vi "Home.vi"() -> ()   [LabVIEW 2019]
uses:
  <vilib>/NI/Current Value Table/Type Defs/Single Tag.ctl
  <vilib>/NI/Current Value Table/Type Defs/Data Types.ctl
  <vilib>/NI/STM/TCP/Read Meta Data (TCP Ref).vi
  <vilib>/NI/STM/TCP/Get Connection Reference (TCP).vi
  <vilib>/NI/AMC/Read Termination Message.vi
  <vilib>/NI/AMC/Create Single Message.vi
  <vilib>/NI/AMC/Update Message Routing Info.vi
  <vilib>/NI/STM/TCP/Read Meta Data (TCP Clst).vi
  <vilib>/NI/AMC/Globals.vi
  <vilib>/NI/STM/TCP/Write Message (TCP).vi
  <vilib>/NI/AMC/Send Message.vi
  <vilib>/NI/AMC/AMC.lvlib
  <vilib>/NI/STM/NI STM.lvlib
  <vilib>/NI/Current Value Table/Current Value Table.lvlib
panel:
  in  "Reset Alarms":bool
  in  "Run":bool
  in  "Alarms":i32(listbox)=-1
  out "PLC Model":string
  out "PLC Firmware":string
  out "PLC Sweep Time":dbl format="%#.4f"
  in  "Exit":bool
  in  "Dosing":bool
  in  "Mixing Tank":bool
  in  "Process 3":bool
  in  "Process 2":bool
  in  "Process 1":bool
  out "status":string
  in  "Home Btn":bool
  in  "Facilities Btn":bool
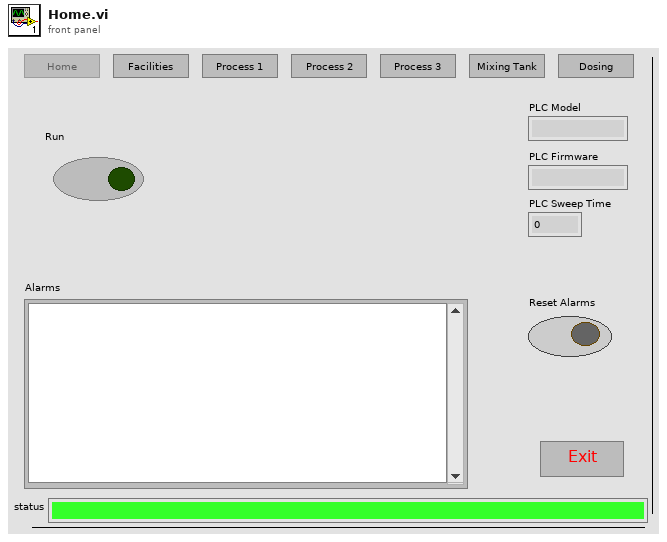
[diagram p1: front panel]
types:
  T1 = typedef "Current Value Table.lvlib/Single Tag.ctl" = cluster{"Data Type":T2, "Name":string, "Value":string, "Description":string}
  T2 = typedef "Current Value Table.lvlib/Data Types.ctl" = enum16{"Double", "Single", "I64", "I32", "I16", "I8", "U64", "U32", "U16", "U8", "String", "Boolean", "Array of U8", "Array of U16", "Array of U32", "Array of U64", "Array of I64", "Array of I32", "Array of I16", "Array of I8", "Array of Double", "Array of Single", "Array of Boolean", "Array of String"}
  T3 = typedef "AMC.lvlib/Message Queue.ctl" = refnum<queue>
  T4 = typedef "NI STM.lvlib/TCP Connection Info.ctl" = cluster{"connection ID":refnum<k5>, "meta data":T5[]}
  T5 = typedef "NI STM.lvlib/MetaDataElement.ctl" = string
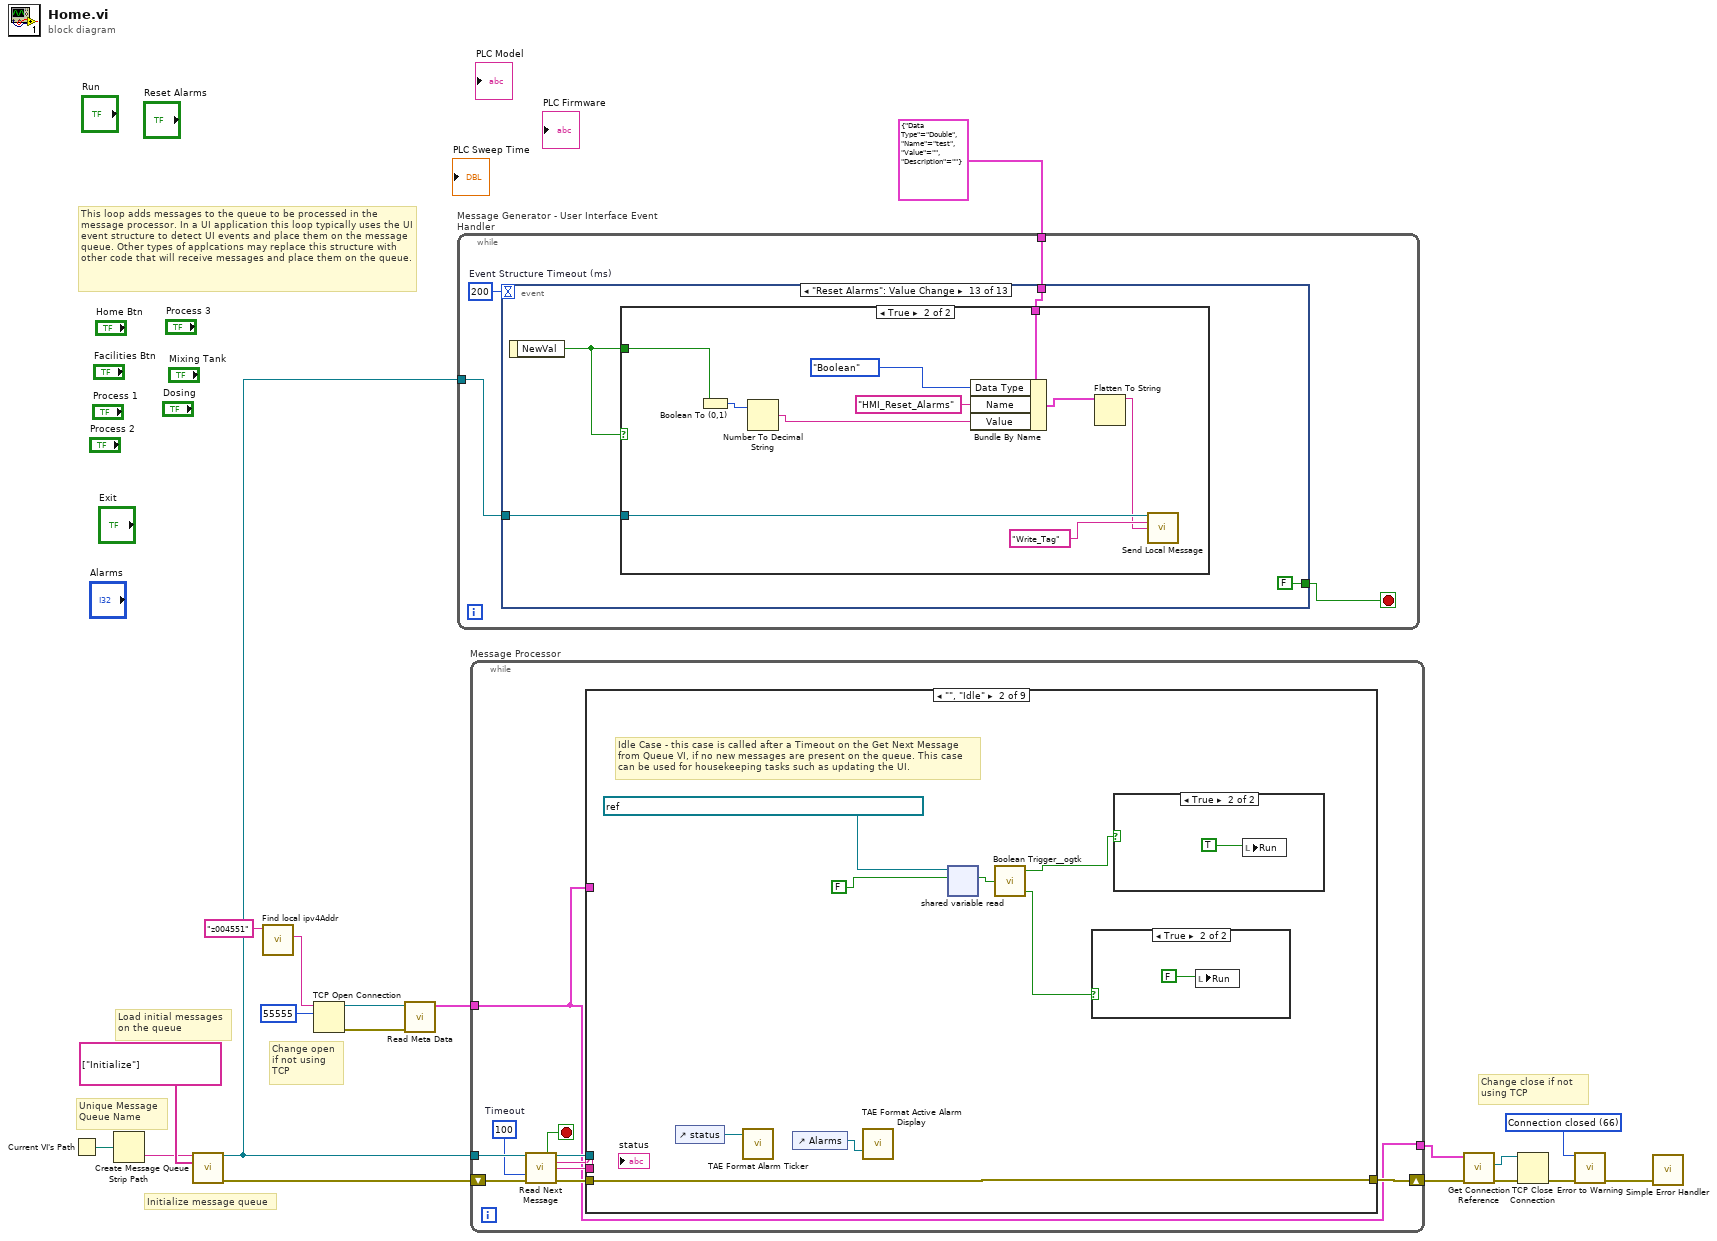
[diagram p0: block diagram]
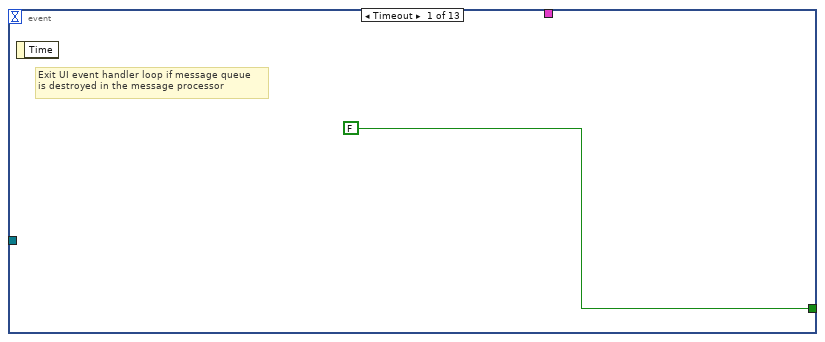
[diagram p2: hidden frame]
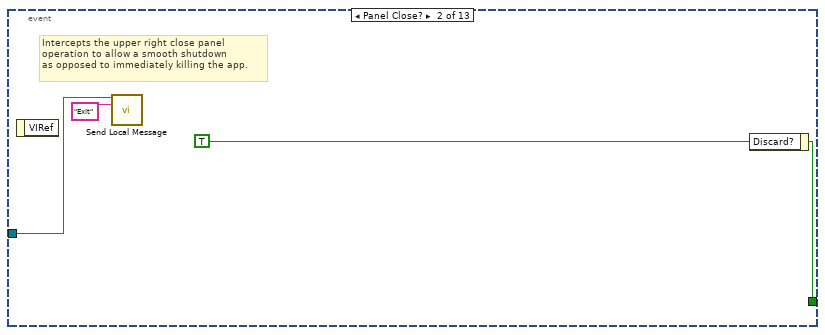
[diagram p3: hidden frame]
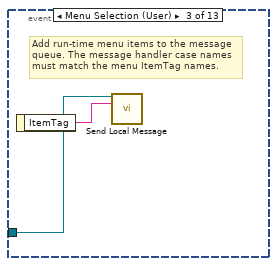
[diagram p4: hidden frame]
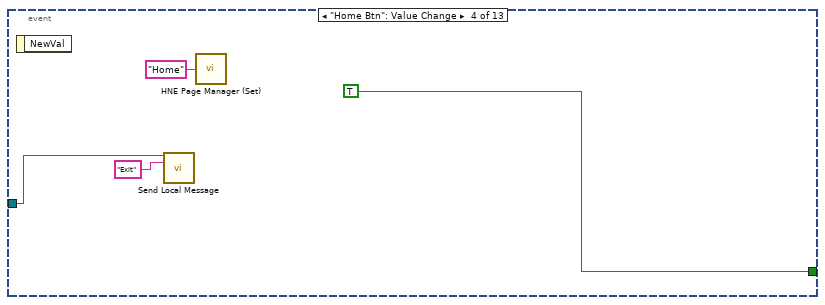
[diagram p5: hidden frame]
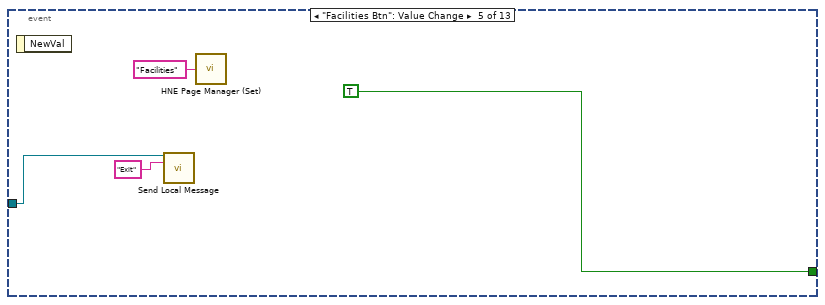
[diagram p6: hidden frame]
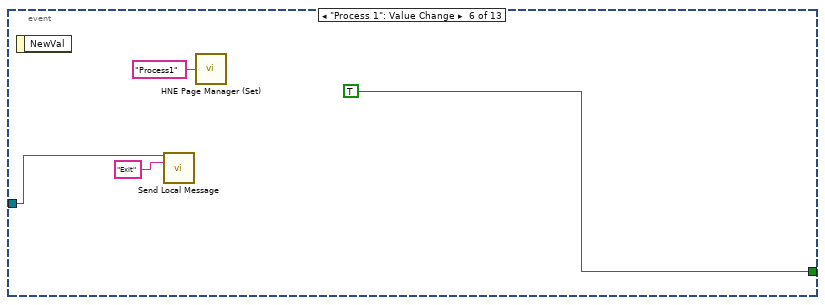
[diagram p7: hidden frame]
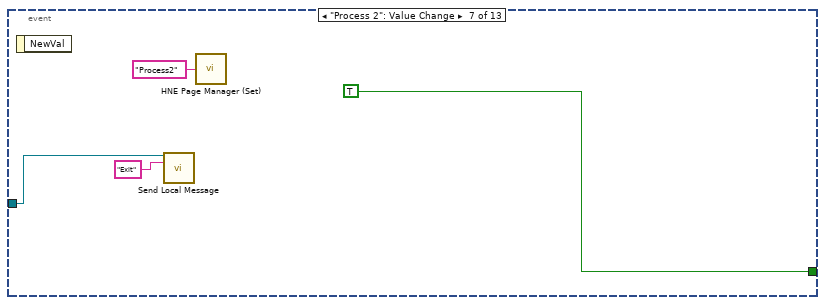
[diagram p8: hidden frame]
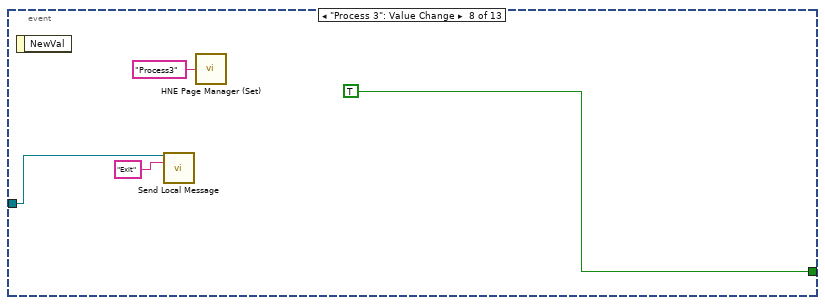
[diagram p9: hidden frame]
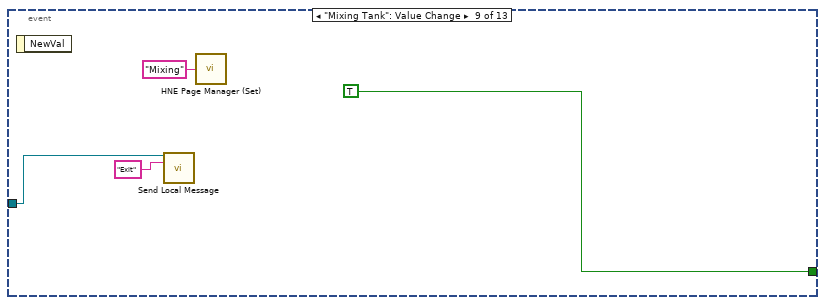
[diagram p10: hidden frame]
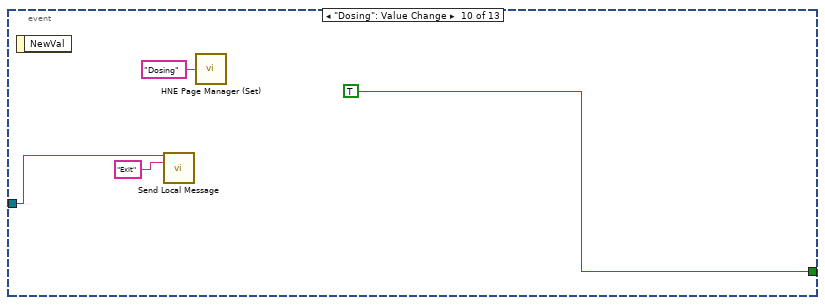
[diagram p11: hidden frame]
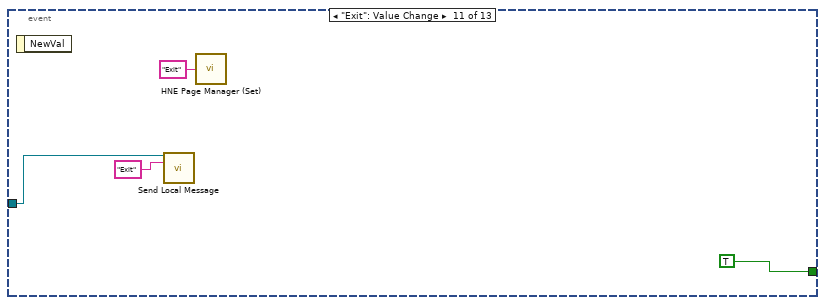
[diagram p12: hidden frame]
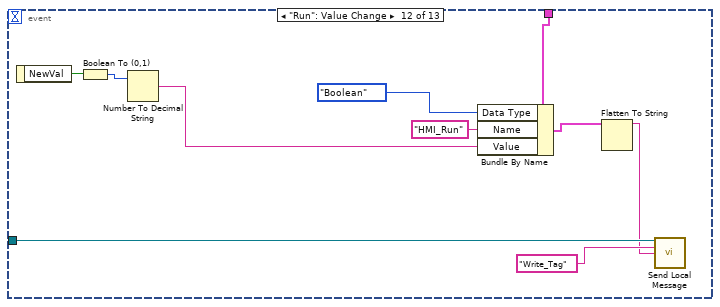
[diagram p13: hidden frame]
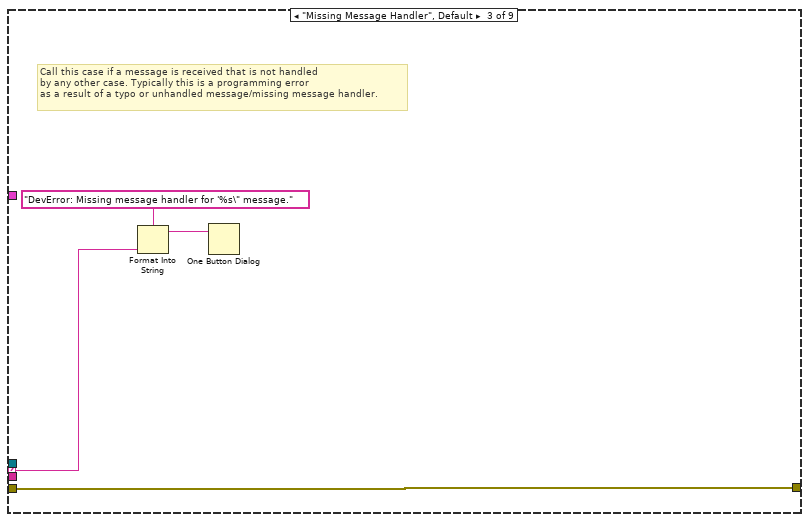
[diagram p18: hidden frame]
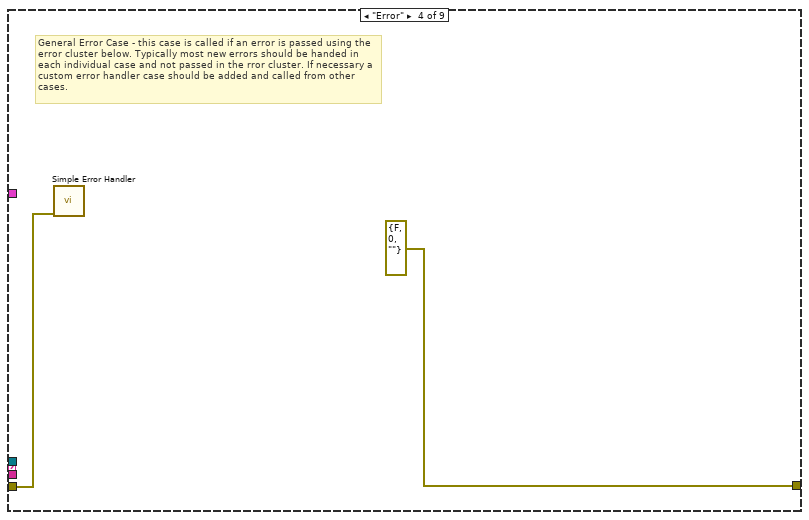
[diagram p19: hidden frame]
diagram:
  w8 = 66 items=["No Error", "Argument Error", "Memory Full", "Out of Zone", "End of File", "File Already Open", "Generic File IO Error", "File Not Found", "File Permission Error", "Disk Full", "Duplicate Path", "Too Many Files Open", "Not Enabled", "Resource File Not Found", "Cannot Add Resource", "Resource Not Found", "Image Not Found", "Image Memory Error", "Pen Does Not Exist", "Config Bad Type", "Config Token Not Found", "Config Parse Error", "Config Memory Error", "Bad External Code Format", "Bad External Code Offset", "External Code Not Present", "Null Window", "Destroy Window Mixup", "Null Menu", "Print Aborted", "Bad Print Record", "Print Driver Error", "Windows Error During Print", "Memory Error During Print", "Print Dialog Error", "Generic Print Error", "Invalid Device Refnum", "Device Not Found", "Device Parameter Error", "Device Unit Error", "Can't Open Device", "Device Call Aborted", "Generic Error", "Cancelled By User", "Object ID Too Low", "Object ID Too High", "Object Not In Heap", "Unknown Heap", "Bad DefProc ID", "DefProc Not In Table", "Message Out Of Range", "Null Method", "Unknown Message", "Manager Call Not Supported", "Bad address", "Connection In progress", "Connection timed out", "Connection is already in progress", "Network attribute not supported", "Network error", "Address in use", "System out of memory", "Connection aborted", "Connection refused", "Connection is not connected", "Connection is already connected", "Connection closed", "Initialize error (interapplication manager)", "Bad occurrence", "Wait on unbound occurrence handler", "Occurrence queue overflow", "Bad path", "Semaphore not signaled", "Unrecognized type (interapplication manager)"] ("1st Error to Convert")
  # "Change close if not using TCP"
  # "Change open if not using TCP"
  # "This loop adds messages to the queue to be processed in the message processor. In a UI application this loop typically uses the UI event structure to detect UI events and place them on the message queue. Other types of applcations may replace this structure with other code that will receive messages and place them on the queue."
  # "Initialize message queue"
  # "Unique Message\nQueue Name"
  # "Load initial messages\non the queue"
  n1 = Current VI's Path() -> (path=w15:path)
  n2 = Strip Path(path=w15) -> (name=w18:string)  [unwired: 1 out]
  n3 = call <vilib>:"Create Message Queue.vi"("message queue name"=w18, "initial message names"=string[] ["Initialize"]) -> ("message queue out"=w17:T3, "error out"=w16:errorcluster)  [unwired: 12 in]
  n4 = call "Find local ipv4Addr.vi"("MachineToFind"="z004551") -> ("name"=w11:string)  [unwired: 9 in, 1 out]
  n5 = TCP Open Connection(address=w11, remote port or service name=u16 55555 ("remote port")) -> (connection ID=w13:refnum<k5>, error out=w12:errorcluster)  [unwired: 1 in, 2 out]
  n6 = call-poly <vilib>:"Read Meta Data.vi"("error in"=w12, "connection ID"=w13) -> ("connection info out"=w3:T4)  [unwired: 7 in, 2 out]
  n7 = while "Message Generator - User Interface Event Handler" {
    tunnel: w17 -> [w21]
    tunnel: T1 {"Data Type"=enum."Double", "Name"="test", "Value"="", "Description"=""} ("Tag") -> [w20]
    stop <- w22 stop-if-true
    w23 = 200  # Event Structure Timeout (ms)
    n8 = event shown="[12] \"Reset Alarms\": Value Change" {
      selector: _ -> [_ _ _ _ _ _ _ _ _ _ _ _ _]
      dyn-events: _ -> [_ _ _ _ _ _ _ _ _ _ _ _ _]
      timeout: w23 -> [_ _ _ _ _ _ _ _ _ _ _ _ _]
      tunnel: [FALSE ("Discard?") w27 _ TRUE ("Discard?") TRUE ("Discard?") TRUE ("Discard?") TRUE ("Discard?") TRUE ("Discard?") TRUE ("Discard?") TRUE ("Discard?") TRUE ("Discard?") _ FALSE ("Discard?")] -> w22
      tunnel: w21 -> [_ w25 w28 w30 w34 w38 w42 w46 w50 w54 w58 w71 w75]
      tunnel: w20 -> [_ _ _ _ _ _ _ _ _ _ _ w67 w74]
      event Timeout {
        # "Exit UI event handler loop if message queue\nis destroyed in the message processor"
        n9 = event-data() -> ()  [unwired: 2 out]
      }
      event Panel Close? {
        w27 = TRUE ("Discard?")
        # "Intercepts the upper right close panel\noperation to allow a smooth shutdown\nas opposed to immediately killing the app."
        n10 = event-data() -> ()  [unwired: 2 out]
        n11 = call <vilib>:"Send Local Message.vi"("message queue in"=w25, "message name"="Exit") -> ()  [unwired: 11 in, 3 out]
        n12 = event-data("Discard?"=w27) -> ()  [unwired: 1 in, 1 out]
      }
      event Menu Selection (User) {
        # "Add run-time menu items to the message\nqueue. The message handler case names must match the menu ItemTag names."
        n13 = event-data() -> ("ItemTag"=w29:string)  [unwired: 1 out]
        n14 = call <vilib>:"Send Local Message.vi"("message queue in"=w28, "message name"=w29) -> ()  [unwired: 11 in, 3 out]
      }
      event "Home Btn": Value Change {
        n15 = event-data() -> ()  [unwired: 2 out]
        n16 = call <vilib>:"Send Local Message.vi"("message queue in"=w30, "message name"="Exit") -> ()  [unwired: 11 in, 3 out]
        n17 = call <userlib>:"HNE Page Manager (Set).vi"("Next Page"="Home") -> ()  [unwired: 4 in, 1 out]
      }
      event "Facilities Btn": Value Change {
        n18 = event-data() -> ()  [unwired: 2 out]
        n19 = call <vilib>:"Send Local Message.vi"("message queue in"=w34, "message name"="Exit") -> ()  [unwired: 11 in, 3 out]
        n20 = call <userlib>:"HNE Page Manager (Set).vi"("Next Page"="Facilities") -> ()  [unwired: 4 in, 1 out]
      }
      event "Process 1": Value Change {
        n21 = event-data() -> ()  [unwired: 2 out]
        n22 = call <vilib>:"Send Local Message.vi"("message queue in"=w38, "message name"="Exit") -> ()  [unwired: 11 in, 3 out]
        n23 = call <userlib>:"HNE Page Manager (Set).vi"("Next Page"="Process1") -> ()  [unwired: 4 in, 1 out]
      }
      event "Process 2": Value Change {
        n24 = event-data() -> ()  [unwired: 2 out]
        n25 = call <vilib>:"Send Local Message.vi"("message queue in"=w42, "message name"="Exit") -> ()  [unwired: 11 in, 3 out]
        n26 = call <userlib>:"HNE Page Manager (Set).vi"("Next Page"="Process2") -> ()  [unwired: 4 in, 1 out]
      }
      event "Process 3": Value Change {
        n27 = event-data() -> ()  [unwired: 2 out]
        n28 = call <vilib>:"Send Local Message.vi"("message queue in"=w46, "message name"="Exit") -> ()  [unwired: 11 in, 3 out]
        n29 = call <userlib>:"HNE Page Manager (Set).vi"("Next Page"="Process3") -> ()  [unwired: 4 in, 1 out]
      }
      event "Mixing Tank": Value Change {
        n30 = event-data() -> ()  [unwired: 2 out]
        n31 = call <vilib>:"Send Local Message.vi"("message queue in"=w50, "message name"="Exit") -> ()  [unwired: 11 in, 3 out]
        n32 = call <userlib>:"HNE Page Manager (Set).vi"("Next Page"="Mixing") -> ()  [unwired: 4 in, 1 out]
      }
      event "Dosing": Value Change {
        n33 = event-data() -> ()  [unwired: 2 out]
        n34 = call <vilib>:"Send Local Message.vi"("message queue in"=w54, "message name"="Exit") -> ()  [unwired: 11 in, 3 out]
        n35 = call <userlib>:"HNE Page Manager (Set).vi"("Next Page"="Dosing") -> ()  [unwired: 4 in, 1 out]
      }
      event "Exit": Value Change {
        n36 = event-data() -> ()  [unwired: 2 out]
        n37 = call <vilib>:"Send Local Message.vi"("message queue in"=w58, "message name"="Exit") -> ()  [unwired: 11 in, 3 out]
        n38 = call <userlib>:"HNE Page Manager (Set).vi"("Next Page"="Exit") -> ()  [unwired: 4 in, 1 out]
      }
      event "Run": Value Change {
        n39 = event-data() -> ("NewVal"=w69:bool)  [unwired: 1 out]
        n40 = Boolean To (0,1)(Boolean=w69) -> (0, 1=w68:i16)
        n41 = Number To Decimal String(number=w68) -> (decimal integer string=w64:string)  [unwired: 1 in]
        n42 = Bundle By Name(cluster=w67, "Data Type"=Data_Types."Boolean", "Name"="HMI_Run", "Value"=w64) -> (w66:T1)
        n43 = Flatten To String(anything=w66) -> (data string=w65:string)  [unwired: 3 in, 2 out]
        n44 = call <vilib>:"Send Local Message.vi"("message queue in"=w71, "message name"="Write_Tag", "message value"=w65) -> ()  [unwired: 10 in, 3 out]
      }
      event "Reset Alarms": Value Change {
        n45 = event-data() -> ("NewVal"=w72:bool)  [unwired: 1 out]
        n46 = case shown="True" w72 {
          tunnel: w75 -> [_ w85]
          tunnel: w72 -> [_ w83]
          tunnel: w74 -> [_ w81]
          frame False {
          }
          frame True {
            n47 = Boolean To (0,1)(Boolean=w83) -> (0, 1=w82:i16)
            n48 = Number To Decimal String(number=w82) -> (decimal integer string=w78:string)  [unwired: 1 in]
            n49 = Bundle By Name(cluster=w81, "Data Type"=Data_Types."Boolean", "Name"="HMI_Reset_Alarms", "Value"=w78) -> (w80:T1)
            n50 = Flatten To String(anything=w80) -> (data string=w79:string)  [unwired: 3 in, 2 out]
            n51 = call <vilib>:"Send Local Message.vi"("message queue in"=w85, "message name"="Write_Tag", "message value"=w79) -> ()  [unwired: 10 in, 3 out]
          }
        }
      }
    }
  }
  n52 = while "Message Processor" {
    shift-left: w16 -> [w91]
    shift-right: [w95] -> w4
    tunnel: w17 -> [w92]
    tunnel: [w86] -> w2
    tunnel: w3 -> [w86]
    stop <- w94 stop-if-true
    w87 = 100  # Timeout
    n53 = call <vilib>:"Read Next Message.vi"("message queue in"=w92, "timeout (1 ms)"=w87, "error in"=w91) -> ("exit process?"=w94:bool, "message queue out"=w93:T3, "message name"=w89:string, "message value"=w88:string, "error out"=w90:errorcluster)  [unwired: 5 in, 3 out]
    n54 = case shown="\"\", \"Idle\"" w89 {
      selector: w89 -> [_ _ w109 _ _ _ _ _ _]
      tunnel: w93 -> [_ _ _ _ _ _ w119 _ _]
      tunnel: w90 -> [w96 w104 w110 w111 w113 w117 w120 w122 w124]
      tunnel: [w96 w104 w110 errorcluster {"status"=FALSE, "code"=0, "source"=""} ("error out") w113 w117 w118 w122 w123] -> w95
      tunnel: w88 -> [_ _ _ _ _ _ _ _ w125]
      tunnel: w86 -> [_ _ _ _ _ _ _ _ w126]
      frame "---------- Framework Operations ----------" {
        # "Dummy case to add a seperator in the Case Structure menu"
      }
      frame "", "Idle" {
        # "Idle Case - this case is called after a Timeout on the Get Next Message from Queue VI, if no new messages are present on the queue. This case can be used for housekeeping tasks such as updating the UI."
        n55 = control-ref of="status"() -> (w103:refnum<vi>)
        n56 = call <userlib>:"TAE Format Alarm Ticker.vi"("Alarm Ticker Ref"=w103) -> ()  [unwired: 15 in]
        n57 = control-ref of="Alarms"() -> (w102:refnum<vi>)
        n58 = call <userlib>:"TAE Format Active Alarm Display.vi"("List Box Ref"=w102) -> ()  [unwired: 14 in, 1 out]
        n59 = shared-variable-read(refnum<k21> "ni.var.psp://z004551/CDL0100 ReadWriteTags/HMI_Run" ("shared variable refnum in"), FALSE) -> (w99:bool)  [unwired: 1 in, 3 out]
        n60 = call <userlib>:"Boolean Trigger__ogtk.vi"("Boolean Input"=w99) -> ("Rising Edge"=w97:bool, "Falling Edge"=w98:bool)  [unwired: 1 in]
        n61 = case shown="True" w98 {
          frame False {
          }
          frame True {
            n62 = local write "Run"(FALSE) -> ()
          }
        }
        n63 = case shown="True" w97 {
          frame False {
          }
          frame True {
            n64 = local write "Run"(TRUE) -> ()
          }
        }
      }
      frame "Missing Message Handler", Default {
        # "Call this case if a message is received that is not handled \nby any other case. Typically this is a programming error\nas a result of a typo or unhandled message/missing message handler."
        n65 = Format Into String(format string="DevError: Missing message handler for '%s\" message." ("message"), w109) -> (resulting string=w107:string)  [unwired: 2 in, 1 out]
        n66 = One Button Dialog(message=w107) -> ()  [unwired: 2 out]
      }
      frame "Error" {
        # "General Error Case - this case is called if an error is passed using the error cluster below. Typically most new errors should be handed in each individual case and not passed in the rror cluster. If necessary a custom error handler case should be added and called from other cases."
        n67 = call <vilib>:"Simple Error Handler.vi"("error in (no error)"=w111) -> ()  [unwired: 1 in, 8 out]
      }
      frame "---------- Generic Operations ----------" {
        # "Dummy case to add a seperator in the Case Structure menu"
      }
      frame "Initialize" {
        # "Initialize the state variables and user interface"
        n68 = shared-variable-read(refnum<k21> "ni.var.psp://z004551/CDL0100 ReadWriteTags/HMI_Run" ("shared variable refnum in"), FALSE) -> (w114:bool)  [unwired: 1 in, 3 out]
        n69 = local write "Run"(w114) -> ()
      }
      frame "Exit" {
        # "Destroy message queue >> this will halt the UI event handler loop"
        # "Stop the VI\n>> Perform any cleanup tasks in this message case.\n>> Clear display before closing."
        n70 = call <vilib>:"Destroy Message Queue.vi"("message queue in"=w119, "error in"=w120) -> ("error out"=w118:errorcluster)  [unwired: 11 in, 2 out]
        n71 = local write "status"("" ("Status")) -> ()
      }
      frame "---------- Application Operations ----------" {
        # "Dummy case to add a seperator in the Case Structure menu"
      }
      frame "Write_Tag" {
        n72 = call-poly <vilib>:"Write Message.vi"("error in"=w124, "data"=w125, "name"="WriteTag", "connection info in"=w126) -> ("error out"=w123:errorcluster)  [unwired: 6 in, 1 out]
      }
    }
  }
  n73 = call-poly <vilib>:"Get Connection Reference.vi"("error in"=w4, "connection info in"=w2) -> ("error out"=w7:errorcluster, "connection ID out"=w6:refnum<k5>)  [unwired: 8 out]
  n74 = TCP Close Connection(connection ID=w6, error in (no error)=w7) -> (error out=w9:errorcluster)  [unwired: 2 out]
  n75 = call <vilib>:"Error to Warning.vi"("1st Error to Convert"=w8, "error in"=w9) -> ("warning out"=w5:errorcluster)  [unwired: 3 in, 10 out]
  n76 = call <vilib>:"Simple Error Handler.vi"("error in (no error)"=w5) -> ()  [unwired: 4 in, 5 out]
